vi "Update OS.vi"(8 "error in (no error)":errorcluster, 11 "RT Management in":refnum<class "RT Management.lvclass">) -> (0 "error out":errorcluster, 1 "Operating System Architecture":string, 2 "Operating System":T1, 3 "RT Management out":refnum<class "RT Management.lvclass">)   [LabVIEW 2016, in "RT Management.lvlib" / "RT Management.lvclass"]
doc: "This VI gets the OS of the RT target and sets the public, read-only \"Operating System\" and \"Operating System Architecture\" properties in the RT Management class. This is a private VI and only intended to be used in the Initialize.vi method since the OS will not change within a single System Configuration API session.\n\nIt also returns the OS of the RT target. The possible values for the \"Operating System\" enum are: Unknown, VxWorks, PharLap, Linux-ARM, and Linux-x64.\n\nThe \"Operating System Architecture\" strings returns the exact string that the System Configuration API returns, even in the case of Unknown."
uses:
  RT Management.lvclass
  Controls/Operating system.ctl
  RT Management.lvclass/RT Management.ctl
  Get SysCfg Session.vi
  Set Operating system.vi
  Set Operating System Architecture.vi
  <resource>/objmgr/nisysapi.rc
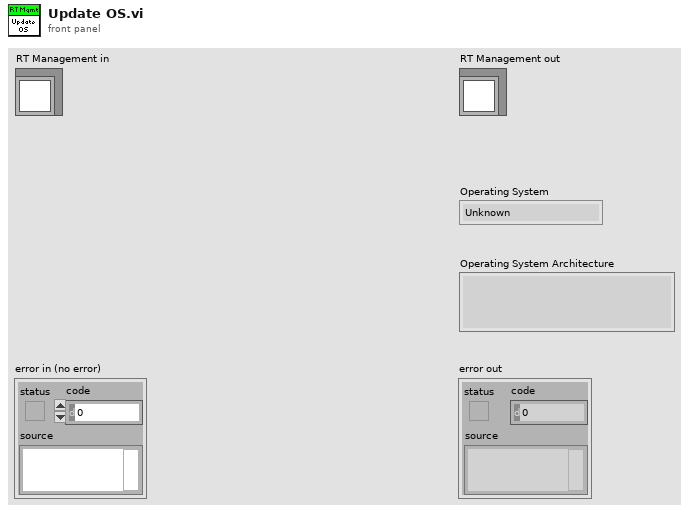
[diagram p1: front panel]
types:
  T1 = typedef "RT Management.lvlib/RT Management.lvclass/Operating system.ctl" = enum16{"Unknown", "VxWorks", "PharLap", "Linux-ARM", "Linux-x64"}
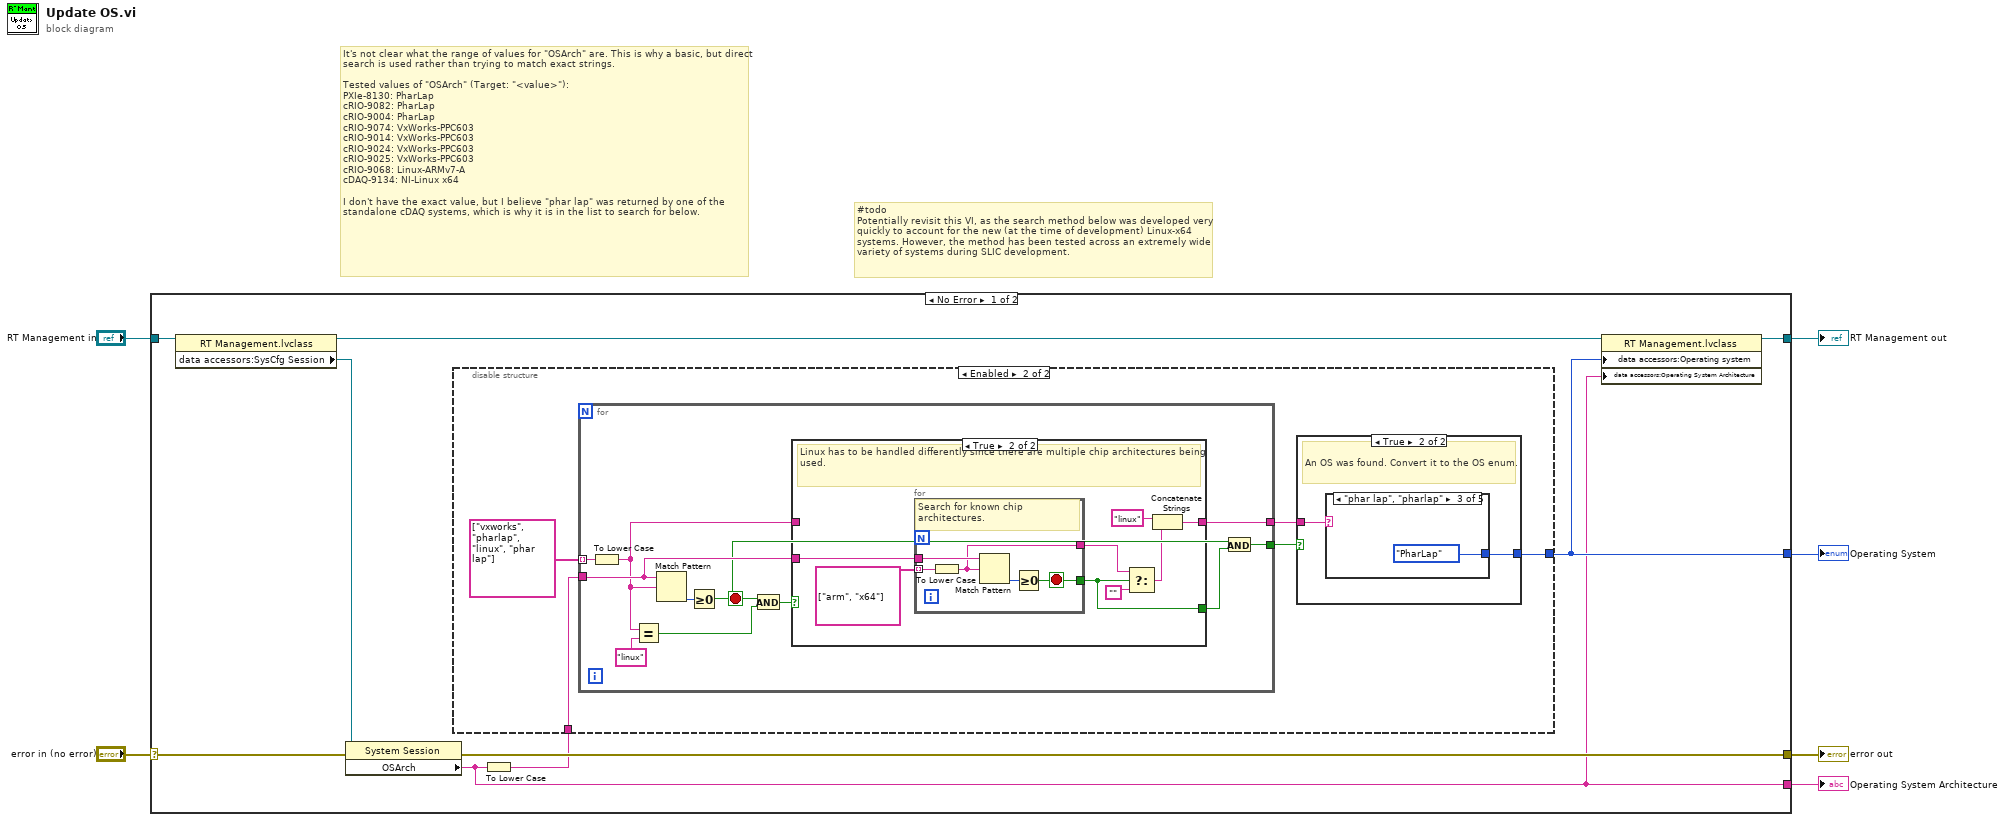
[diagram p0: block diagram]
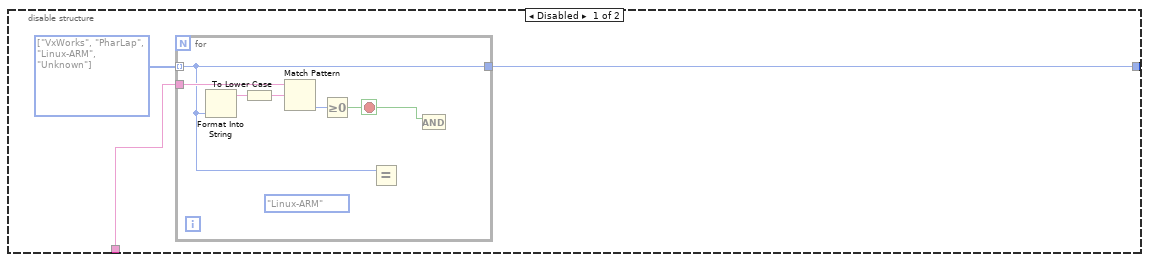
[diagram p2: hidden frame]
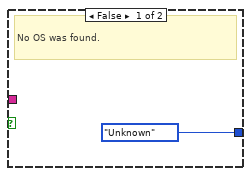
[diagram p3: hidden frame]
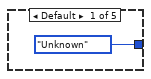
[diagram p4: hidden frame]
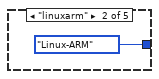
[diagram p5: hidden frame]
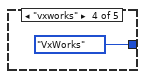
[diagram p6: hidden frame]
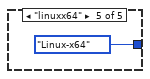
[diagram p7: hidden frame]
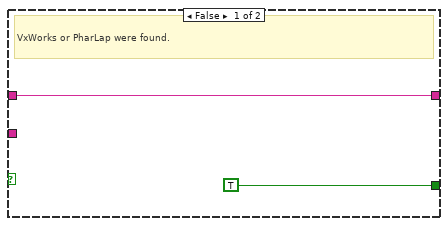
[diagram p8: hidden frame]
diagram:
  # "#todo\nPotentially revisit this VI, as the search method below was developed very quickly to account for the new (at the time of development) Linux-x64 systems. However, the method has been tested across an extremely wide variety of systems during SLIC development."
  # "It's not clear what the range of values for \"OSArch\" are. This is why a basic, but direct search is used rather than trying to match exact strings.\n\nTested values of \"OSArch\" (Target: \"<value>\"):\nPXIe-8130: PharLap\ncRIO-9082: PharLap\ncRIO-9004: PharLap\ncRIO-9074: VxWorks-PPC603\ncRIO-9014: VxWorks-PPC603\ncRIO-9024: VxWorks-PPC603\ncRIO-9025: VxWorks-PPC603\ncRIO-9068: Linux-ARMv7-A\ncDAQ-9134: NI-Linux x64\n\nI don't have the exact value, but I believe \"phar lap\" was returned by one of the standalone cDAQ systems, which is why it is in the list to search for below."
  n1 = case shown="No Error" "error in (no error)" {
    selector: "error in (no error)" -> [w14 w65]
    tunnel: [w13 w65] -> w5
    tunnel: [w9 w64] -> w3
    tunnel: "RT Management in" -> [w15 w64]
    tunnel: [w8 _] -> w2
    tunnel: [w7 _] -> w1
    frame No Error {
      n2 = property class="RT Management.lvclass"(reference=w15) -> (reference out=w10:refnum<class "RT Management.lvclass">, "data accessors:SysCfg Session"=w12:refnum<k21>)  [unwired: 1 in, 1 out]
      n3 = property class="System Session"(reference=w12, error in=w14) -> (error out=w13:errorcluster, "OSArch"=w7:string)  [unwired: 1 out]
      n4 = To Lower Case(string=w7) -> (all lower case string=w11:string)
      n5 = disable-structure shown="Enabled" {
        disable-tunnel: w11 -> [w16 w26]
        disable-tunnel: [w17 w25] -> w8
        frame Disabled {
          w18 = T1[] [enum."VxWorks", enum."PharLap", enum."Linux-ARM", enum."Unknown"] items=["Unknown", "VxWorks", "PharLap", "Linux-ARM", "Linux-x64"]
          n6 = for {
            tunnel: w16 -> [w23]
            tunnel: w18 -> [w19] mode=indexing
            tunnel: [w19] -> w17
            stop <- w20 stop-if-true
            (unwired) Operating_system."Linux-ARM" ("y")
            n7 = Format Into String(w19) -> (resulting string=w22:string)  [unwired: 3 in, 1 out]
            n8 = To Lower Case(string=w22) -> (all lower case string=w21:string)
            n9 = Match Pattern(string=w23, regular expression=w21) -> (offset past match=w24:i32)  [unwired: 1 in, 3 out]
            n10 = Greater Or Equal To 0?(x=w24) -> (x >= 0?=w20:bool)
            n11 = Equal?(x=w19) -> ()  [unwired: 1 in, 1 out]
            n12 = And(x=w20) -> ()  [unwired: 1 in, 1 out]
          }
        }
        frame Enabled {
          n13 = for {
            tunnel: w26 -> [w40]
            tunnel: string[] ["vxworks", "pharlap", "linux", "phar lap"] -> [w47] mode=indexing
            tunnel: [w42] -> w28
            tunnel: [w41] -> w29
            stop <- w38 stop-if-true
            # "Determine what"
            n14 = To Lower Case(string=w47) -> (all lower case string=w39:string)
            n15 = Equal?(x=w39, y="linux") -> (x = y?=w45:bool)
            n16 = Match Pattern(string=w40, regular expression=w39) -> (offset past match=w48:i32)  [unwired: 1 in, 3 out]
            n17 = Greater Or Equal To 0?(x=w48) -> (x >= 0?=w38:bool)
            n18 = And(x=w38, y=w45) -> (x .and. y?=w44:bool)
            n19 = case shown="True" w44 {
              tunnel: w40 -> [_ w58]
              tunnel: [TRUE w56] -> w43
              tunnel: [w49 w51] -> w41
              tunnel: w39 -> [w49 _]
              frame False {
                # "VxWorks or PharLap were found."
              }
              frame True {
                # "Linux has to be handled differently since there are multiple chip architectures being used."
                n20 = for {
                  tunnel: w58 -> [w60]
                  tunnel: string[] ["arm", "x64"] -> [w63] mode=indexing
                  tunnel: [w61] -> w56
                  tunnel: [w59] -> w55
                  stop <- w61 stop-if-true
                  # "Search for known chip architectures."
                  n21 = To Lower Case(string=w63) -> (all lower case string=w59:string)
                  n22 = Match Pattern(string=w60, regular expression=w59) -> (offset past match=w62:i32)  [unwired: 1 in, 3 out]
                  n23 = Greater Or Equal To 0?(x=w62) -> (x >= 0?=w61:bool)
                }
                n24 = Select(t=w55, s=w56, f="") -> (s? t:f=w53:string)
                n25 = Concatenate Strings("linux" ("string"), w53) -> (w51:string)
              }
            }
            n26 = And(x=w38, y=w43) -> (x .and. y?=w42:bool)
          }
          n27 = case shown="True" w28 {
            tunnel: [Operating_system."Unknown" ("Operating System") w31] -> w25
            tunnel: w29 -> [_ w32]
            frame False {
              # "No OS was found."
            }
            frame True {
              # "An OS was found. Convert it to the OS enum."
              n28 = case shown="\"phar lap\", \"pharlap\"" w32 {
                tunnel: [Operating_system."Unknown" ("Operating System") Operating_system."Linux-ARM" ("Operating System") Operating_system."PharLap" ("Operating System") Operating_system."VxWorks" ("Operating System") Operating_system."Linux-x64" ("Operating System")] -> w31
                frame Default {
                }
                frame "linuxarm" {
                }
                frame "phar lap", "pharlap" {
                }
                frame "vxworks" {
                }
                frame "linuxx64" {
                }
              }
            }
          }
        }
      }
      n29 = property class="RT Management.lvclass"(reference=w10, "data accessors:Operating system"=w8, "data accessors:Operating System Architecture"=w7) -> (reference out=w9:refnum<class "RT Management.lvclass">)  [unwired: 1 in, 1 out]
    }
    frame Error {
    }
  }
  "error out" <- w5
  "RT Management out" <- w3
  "Operating System" <- w2
  "Operating System Architecture" <- w1
